vi "Create Volatus Group.vi"(7 "Group Type (Abstract)":refnum<class "GroupAbstract.lvclass">, 8 "error in (no error)":errorcluster, 10 "Volatus Group":refnum<class "Group.lvclass">, 11 "TelemetryAPI":refnum<class "TelemetryAPI.lvclass">) -> (0 "error out":errorcluster, 2 "Group":refnum<class "GroupAbstract.lvclass">)   [LabVIEW 2020, in "Volatus.lvlib"]
uses:
  Volatus.lvlib
  VolatusConfig/Group/Group.lvclass
  VolatusConfig/Channel/Channel.lvclass
  TelemetryAPI/TelemetryAPI.lvclass
  lv-vecto/Vecto/Publish Config.ctl
  lv-vecto/Vecto/Vecto.lvlib
  lv-vecto/Vecto/Group/Group.lvclass
  lv-vecto/Vecto/StringGroup/StringGroup.lvclass
  C:/dev/lv20CE/relink/lv-volatus/VolatusConfig/VolatusConfigElement/VolatusConfigElement.lvclass
  C:/dev/lv20CE/relink/lv-volatus/VolatusConfig/Channel/Channel.lvclass
  VolatusConfig/VolatusConfigElement/VolatusConfigElement.lvclass
  C:/dev/lv20CE/relink/lv-vecto/Vecto/GroupAbstract/GroupAbstract.lvclass
  C:/dev/lv20CE/relink/lv-vecto/Vecto/Group/Group.lvclass
  C:/dev/lv20CE/relink/lv-vecto/Vecto/StringGroup/StringGroup.lvclass
  lv-vecto/Vecto/GroupAbstract/GroupAbstract.lvclass
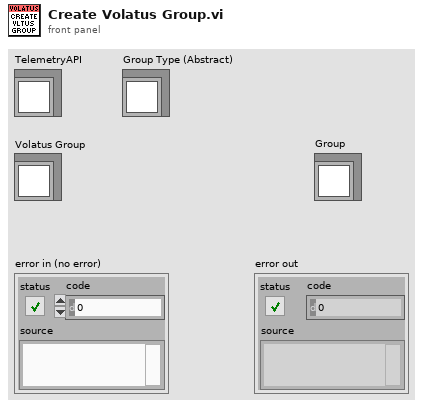
[diagram p1: front panel]
types:
  T1 = typedef "Vecto.lvlib/Publish Config.ctl" = cluster{"Address":string, "Port":u16}
  T2 = typedef "Vecto.lvlib/Group Info.ctl" = cluster{"System":string, "Cluster":string, "Node":string, "Task":string, "Name":string}
  T3 = typedef "VolatusConfig.lvlib/Endpoint.ctl" = cluster{"Address":string, "Port":u16}
  T4 = typedef "VolatusConfig.lvlib/Group Type.ctl" = enum16{"Double", "String"}
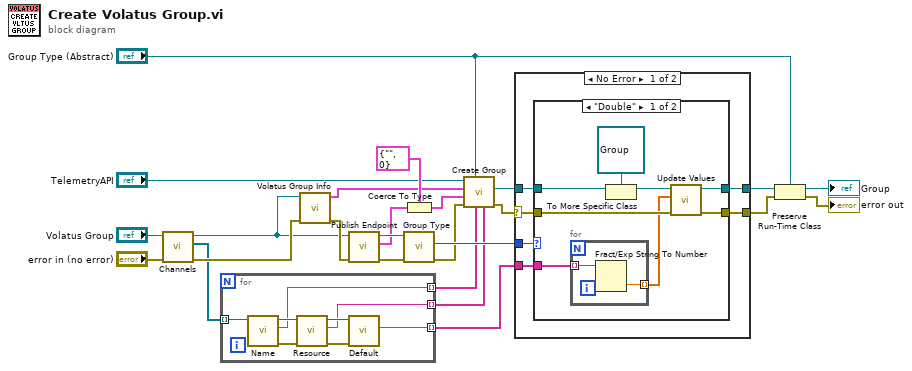
[diagram p0: block diagram]
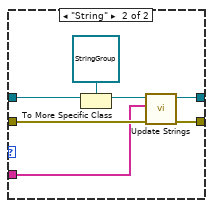
[diagram p2: hidden frame]
diagram:
  n1 = call "Channels.vi"("error in (no error)"="error in (no error)", "Group in"="Volatus Group") -> ("error out"=w23:errorcluster, "Channels"=w21:refnum<class "Channel.lvclass">[], "Group out"=w17:refnum<class "Group.lvclass">)  [unwired: 7 in]
  n2 = for {
    tunnel: w21 -> [w33] mode=indexing
    tunnel: [w28] -> w20 mode=indexing
    tunnel: [w27] -> w7 mode=indexing
    tunnel: [w26] -> w8 mode=indexing
    n3 = call "Name.vi"("VolatusConfigElement in"=w33) -> ("error out"=w31:errorcluster, "Name"=w27:string, "VolatusConfigElement out"=w32:refnum<class "Channel.lvclass">)  [unwired: 8 in]
    n4 = call "Resource.vi"("error in (no error)"=w31, "Channel in"=w32) -> ("error out"=w29:errorcluster, "Resource"=w26:string, "Channel out"=w30:refnum<class "Channel.lvclass">)  [unwired: 7 in]
    n5 = call "Default.vi"("error in (no error)"=w29, "Channel in"=w30) -> ("Default"=w28:string)  [unwired: 7 in, 2 out]
  }
  n6 = call "Volatus Group Info.vi"("error in (no error)"=w23, "Volatus Group"=w17) -> ("error out"=w24:errorcluster, "Group Info"=w4:T2)  [unwired: 8 in]
  n7 = call "Publish Endpoint.vi"("error in (no error)"=w24, "Group in"=w17) -> ("error out"=w25:errorcluster, "Publish Endpoint"=w11:T3, "Group out"=w18:refnum<class "Group.lvclass">)  [unwired: 7 in]
  n8 = Coerce To Type(0:w11, 1:T1 {"Address"="", "Port"=0} ("Publish Config (None)")) -> (2:w5:T1)
  n9 = call "Group Type.vi"("error in (no error)"=w25, "Group in"=w18) -> ("error out"=w6:errorcluster, "Group Type"=w19:T4)  [unwired: 7 in, 1 out]
  n10 = call "Create Group.vi"("Channel Resources (Unset)"=w8, "Channel Names"=w7, "Group Type"="Group Type (Abstract)", "error in (no error)"=w6, "Publish Config (None)"=w5, "Group Info"=w4, "TelemetryAPI in"="TelemetryAPI") -> ("error out"=w2:errorcluster, "Group"=w1:refnum<class "GroupAbstract.lvclass">)  [unwired: 2 in, 1 out]
  n11 = case shown="No Error" w2 {
    selector: w2 -> [w35 w57]
    tunnel: w20 -> [w39 _]
    tunnel: w19 -> [w38 _]
    tunnel: [w37 _] -> w15
    tunnel: [w36 w57] -> w14
    tunnel: w1 -> [w34 _]
    frame No Error {
      n12 = case shown="\"Double\"" w38 {
        tunnel: w39 -> [w47 w50]
        tunnel: [w46 w56] -> w36
        tunnel: [w45 w55] -> w37
        tunnel: w35 -> [w44 w54]
        tunnel: w34 -> [w43 w53]
        frame "Double" {
          n13 = for {
            tunnel: w47 -> [w49] mode=indexing
            tunnel: [w48] -> w40 mode=indexing
            n14 = Fract/Exp String To Number(string=w49) -> (number=w48:dbl)  [unwired: 3 in, 1 out]
          }
          n15 = To More Specific Class(target class=refnum<class "Group.lvclass"> refnum ("Vecto.lvlib:Group.lvclass"), reference=w43) -> (specific class reference=w42:refnum<class "Group.lvclass">)  [unwired: 1 in, 1 out]
          n16 = call "Update Values.vi"("error in (no error)"=w44, "Values"=w40, "Group in"=w42) -> ("error out"=w46:errorcluster, "Group out"=w45:refnum<class "Group.lvclass">)  [unwired: 7 in]
        }
        frame "String" {
          n17 = To More Specific Class(target class=refnum<class "StringGroup.lvclass"> refnum ("Vecto.lvlib:StringGroup.lvclass"), reference=w53) -> (specific class reference=w52:refnum<class "StringGroup.lvclass">)  [unwired: 1 in, 1 out]
          n18 = call "Update Strings.vi"("error in (no error)"=w54, "Strings"=w50, "StringGroup in"=w52) -> ("error out"=w56:errorcluster, "StringGroup out"=w55:refnum<class "StringGroup.lvclass">)  [unwired: 7 in]
        }
      }
    }
    frame Error {
    }
  }
  n19 = Preserve Run-Time Class(object in=w15, error in=w14, 2:"Group Type (Abstract)") -> (object out=→"Group":refnum<class "GroupAbstract.lvclass">, error out=→"error out":errorcluster)
